vi "TimeString.vi"() -> (3 "String":string)   [LabVIEW 2011]
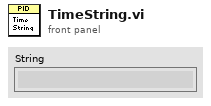
[diagram p1: front panel]
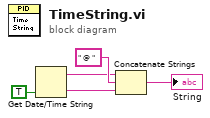
[diagram p0: block diagram]
diagram:
  n1 = Get Date/Time String(want seconds? (F)=TRUE) -> (date string=w1:string, time string=w2:string)  [unwired: 2 in]
  n2 = Concatenate Strings(w1, " @ " ("string"), w2) -> (→"String":string)
